vi "Esperienza 5 TEST 4F 4 paper.vi"() -> ()   [LabVIEW 2019]
uses:
  <vilib>/Analysis/baseanly.llb/Mean (DBL).vi
  <vilib>/Instr/_visa.llb/VISA Configure Serial Port (Instr).vi
  <vilib>/Utility/file.llb/Write Delimited Spreadsheet (DBL).vi
  <vilib>/Analysis/NI_AALBase.lvlib
panel:
  out "Ongoing":bool
  in  "IV":bool
  in  "Set Temperature Temperature":bool
  in  "Temperature Set":dbl=25.0 min=25.0 max=70.0 format="%#_6p"
  out "Actual temperature":dbl=25.0211735 caption="Temperature" format="%#.2g"
  out "V2":dbl[](graph)
  out "V1":dbl[](graph)
  out "V0":dbl[](graph)
  out "V2":dbl[](array[numeric])
  out "V1":dbl[](array[numeric])
  out "V0":dbl[](array[numeric])
  in  "R":dbl=10.0 format="%#_6p"
  out "Stabilization time":u8(slide)=3 scale=0.0..100.0
  in  "Skip stabilization?":bool
  in  "ITC ON?":bool=TRUE
  in  "Correction":i32=3000 min=0 max=4095 step=1
  in  "LED OP":u16(ring) items=["0.25 sun", "0.5 sun", "0.75 sun", "1 sun"]
  in  "number":i32=4095
  out "Actual current":dbl=0.005 caption="Temperature" format="%#_6p"
  out "Set":bool
  out "read buffer 2":string
  in  "File Name":string="Device 2.7"
  in  "file path":path=path "C:/Users/root/Desktop/Test Didattica Celle"
  in  "Save":bool
  in  "VISA ITC4005":refnum<visa-resource-name>="USB0::0x1313::0x804A::M00320668::INSTR" caption="resource name"
  out "IV Graph":cluster{"Y":dbl[], "Y":dbl[]}[](graph)=[{"Y"=[0.012, 0.023, 0.032, 0.044, 0.052, 0.068, 0.077, 0.085, 0.097, 0.108, 0.12, 0.131, 0.143, 0.152, 0.162, 0.175, 0.182, 0.196, 0.203, 0.218, 0.225, 0.24, 0.249, 0.259, 0.269, 0.281, 0.295, 0.302, 0.315, 0.322, 0.338, 0.348, 0.357, 0.367, 0.38, 0.39, 0.4, 0.409, 0.422, 0.433, 0.443, 0.453, 0.467, 0.476, 0.488, 0.496, 0.508, 0.518, 0.528, 0.537, 0.55, 0.559, 0.572, 0.582, 0.596, 0.6, 0.615, 0.623, 0.636, 0.648, 0.661, 0.67, 0.676, 0.691, 0.7, 0.716, 0.724, 0.732, 0.75, 0.753, 0.767, 0.778, 0.788, 0.799, 0.809, 0.82, 0.832, 0.843, 0.853, 0.862, 0.876, 0.885, 0.895, 0.905, 0.915, 0.929, 0.938, 0.95, 0.962, 0.973, 0.979, 0.99, 1.004, 1.012, 1.024, 1.035, 1.048, 1.058, 1.069, 1.077, 1.086, 1.098, 1.11, 1.12, 1.133, 1.144, 1.154, 1.161, 1.176, 1.184, 1.198, 1.207, 1.214, 1.227, 1.238, 1.248, 1.259, 1.273, 1.283, 1.293, 1.303, 1.315, 1.326, 1.335, 1.348, 1.356, 1.37, 1.378, 1.391, 1.401, 1.411, 1.421, 1.434, 1.443, 1.455, 1.464, 1.476, 1.487, 1.499, 1.509, 1.519, 1.53, 1.541, 1.551, 1.563, 1.572, 1.584, 1.596, 1.605, 1.615, 1.626, 1.638, 1.648, 1.657, 1.67, 1.68, 1.69, 1.701, 1.713, 1.722, 1.734, 1.744, 1.756, 1.766, 1.777, 1.787, 1.798, 1.809, 1.82, 1.831, 1.841, 1.852, 1.862, 1.873, 1.884, 1.895, 1.905, 1.917, 1.927, 1.937, 1.949, 1.958, 1.969, 1.979, 1.986, 1.99, 1.995, 1.999, 2.001, 2.006, 2.009, 2.013, 2.015, 2.018, 2.019, 2.023, 2.026, 2.027, 2.028, 2.032, 2.033, 2.035, 2.037, 2.038, 0.0], "Y"=[0.16, -0.08, -0.32, -0.24, 0.08, -0.08, 0.0, 0.0, 0.0, 0.0, 0.0, -0.16, -0.32, -0.08, -0.08, 0.0, 0.16, 0.0, 0.32, -0.24, 0.0, -0.24, -0.08, 0.08, 0.0, 0.0, -0.16, 0.08, -0.16, 0.32, 0.0, 0.32, 0.0, 0.16, -0.16, 0.16, 0.0, 0.4, 0.08, 0.24, 0.4, 0.08, 0.0, 0.0, 0.08, 0.24, 0.08, 0.0, 0.08, 0.24, 0.0, 0.24, 0.16, 0.24, -0.08, 0.48, 0.16, 0.24, 0.08, 0.24, 0.16, 0.08, 0.56, 0.24, 0.08, 0.16, 0.24, 0.24, -0.16, 0.32, 0.0, -0.16, 0.16, 0.16, 0.16, 0.32, 0.0, 0.16, 0.0, 0.24, 0.16, 0.16, 0.32, 0.48, 0.32, 0.16, 0.16, 0.08, 0.16, 0.24, 0.48, 0.48, 0.32, 0.4, 0.24, 0.16, 0.08, 0.24, 0.16, 0.48, 0.32, 0.56, 0.16, 0.48, 0.4, 0.16, 0.4, 0.48, 0.24, 0.48, 0.32, 0.56, 0.56, 0.64, 0.73, 0.81, 0.73, 0.73, 0.81, 0.64, 0.81, 1.05, 0.89, 0.81, 0.89, 0.97, 0.97, 1.05, 0.97, 1.21, 1.21, 1.13, 1.29, 1.45, 1.45, 1.53, 1.53, 1.53, 1.45, 1.61, 1.69, 1.77, 1.69, 1.85, 2.01, 2.01, 2.1, 2.18, 2.26, 2.42, 2.5, 2.58, 2.66, 2.66, 2.9, 2.9, 3.14, 3.14, 3.3, 3.3, 3.55, 3.63, 3.87, 4.03, 4.27, 4.43, 4.59, 4.59, 4.92, 5.0, 5.4, 5.56, 5.88, 6.12, 6.45, 6.77, 7.17, 7.41, 7.9, 8.22, 8.62, 9.11, 9.67, 9.91, 10.32, 10.64, 10.88, 11.12, 11.36, 11.52, 11.68, 11.85, 12.01, 12.25, 12.33, 12.57, 12.65, 12.81, 12.97, 13.05, 13.3, 13.46, 13.54, 13.7]}]
  out "I":dbl[](array[numeric])=[0.16, -0.08, -0.32, -0.24, 0.08, -0.08, 0.0, 0.0, 0.0, 0.0, 0.0, -0.16, -0.32, -0.08, -0.08, 0.0, 0.16, 0.0, 0.32, -0.24, 0.0, -0.24, -0.08, 0.08, 0.0, 0.0, -0.16, 0.08, -0.16, 0.32, 0.0, 0.32, 0.0, 0.16, -0.16, 0.16, 0.0, 0.4, 0.08, 0.24, 0.4, 0.08, 0.0, 0.0, 0.08, 0.24, 0.08, 0.0, 0.08, 0.24, 0.0, 0.24, 0.16, 0.24, -0.08, 0.48, 0.16, 0.24, 0.08, 0.24, 0.16, 0.08, 0.56, 0.24, 0.08, 0.16, 0.24, 0.24, -0.16, 0.32, 0.0, -0.16, 0.16, 0.16, 0.16, 0.32, 0.0, 0.16, 0.0, 0.24, 0.16, 0.16, 0.32, 0.48, 0.32, 0.16, 0.16, 0.08, 0.16, 0.24, 0.48, 0.48, 0.32, 0.4, 0.24, 0.16, 0.08, 0.24, 0.16, 0.48, 0.32, 0.56, 0.16, 0.48, 0.4, 0.16, 0.4, 0.48, 0.24, 0.48, 0.32, 0.56, 0.56, 0.64, 0.73, 0.8100000000000002, 0.73, 0.73, 0.8100000000000002, 0.64, 0.8100000000000002, 1.05, 0.89, 0.8100000000000002, 0.89, 0.97, 0.97, 1.05, 0.97, 1.21, 1.21, 1.13, 1.29, 1.45, 1.45, 1.53, 1.53, 1.53, 1.45, 1.61, 1.69, 1.77, 1.69, 1.85, 2.01, 2.01, 2.1, 2.18, 2.26, 2.42, 2.5, 2.58, 2.66, 2.66, 2.9, 2.9, 3.14, 3.14, 3.3, 3.3, 3.55, 3.63, 3.87, 4.03, 4.27, 4.43, 4.59, 4.59, 4.92, 5.0, 5.4, 5.56, 5.88, 6.12, 6.45, 6.769999999999999, 7.17, 7.409999999999999, 7.9, 8.22, 8.62, 9.11, 9.67, 9.91, 10.32, 10.64, 10.88, 11.12, 11.36, 11.52, 11.68, 11.85, 12.01, 12.25, 12.33, 12.57, 12.65, 12.809999999999999, 12.970000000000002, 13.05, 13.3, 13.460000000000003, 13.539999999999997, 13.7]
  out "V":dbl[](array[numeric])=[0.012, 0.023, 0.032, 0.044, 0.052, 0.068, 0.077, 0.085, 0.097, 0.108, 0.12, 0.131, 0.143, 0.152, 0.162, 0.175, 0.182, 0.196, 0.203, 0.218, 0.225, 0.24, 0.249, 0.259, 0.269, 0.281, 0.295, 0.302, 0.315, 0.322, 0.338, 0.348, 0.357, 0.367, 0.38, 0.39, 0.4, 0.409, 0.422, 0.433, 0.443, 0.453, 0.467, 0.476, 0.488, 0.496, 0.508, 0.518, 0.528, 0.537, 0.55, 0.559, 0.572, 0.582, 0.596, 0.6, 0.615, 0.623, 0.636, 0.648, 0.661, 0.67, 0.676, 0.691, 0.7, 0.716, 0.724, 0.732, 0.75, 0.753, 0.767, 0.778, 0.788, 0.799, 0.809, 0.82, 0.832, 0.843, 0.853, 0.862, 0.876, 0.885, 0.895, 0.905, 0.915, 0.929, 0.938, 0.95, 0.962, 0.973, 0.979, 0.99, 1.004, 1.012, 1.024, 1.035, 1.048, 1.058, 1.069, 1.077, 1.086, 1.098, 1.11, 1.12, 1.133, 1.144, 1.154, 1.161, 1.176, 1.184, 1.198, 1.207, 1.214, 1.227, 1.238, 1.248, 1.259, 1.273, 1.283, 1.293, 1.303, 1.315, 1.326, 1.335, 1.348, 1.356, 1.37, 1.378, 1.391, 1.401, 1.411, 1.421, 1.434, 1.443, 1.455, 1.464, 1.476, 1.487, 1.499, 1.509, 1.519, 1.53, 1.541, 1.551, 1.563, 1.572, 1.584, 1.596, 1.605, 1.615, 1.626, 1.638, 1.648, 1.657, 1.67, 1.68, 1.69, 1.701, 1.713, 1.722, 1.734, 1.744, 1.756, 1.766, 1.777, 1.787, 1.798, 1.809, 1.82, 1.831, 1.841, 1.852, 1.862, 1.873, 1.884, 1.895, 1.905, 1.917, 1.927, 1.937, 1.949, 1.958, 1.969, 1.979, 1.986, 1.99, 1.995, 1.999, 2.001, 2.006, 2.009, 2.013, 2.015, 2.018, 2.019, 2.023, 2.026, 2.027, 2.028, 2.032, 2.033, 2.035, 2.037, 2.038, 0.0]
  out "array":dbl[](array[numeric])=[0.053, 0.08, 0.012, 0.16, 0.023, -0.08, 0.032, -0.32, 0.044, -0.24, 0.052, 0.08, 0.068, -0.08, 0.077, 0.0, 0.085, 0.0, 0.097, 0.0, 0.108, 0.0, 0.12, 0.0, 0.131, -0.16, 0.143, -0.32, 0.152, -0.08, 0.162, -0.08, 0.175, 0.0, 0.182, 0.16, 0.196, 0.0, 0.203, 0.32, 0.218, -0.24, 0.225, 0.0, 0.24, -0.24, 0.249, -0.08, 0.259, 0.08, 0.269, 0.0, 0.281, 0.0, 0.295, -0.16, 0.302, 0.08, 0.315, -0.16, 0.322, 0.32, 0.338, 0.0, 0.348, 0.32, 0.357, 0.0, 0.367, 0.16, 0.38, -0.16, 0.39, 0.16, 0.4, 0.0, 0.409, 0.4, 0.422, 0.08, 0.433, 0.24, 0.443, 0.4, 0.453, 0.08, 0.467, 0.0, 0.476, 0.0, 0.488, 0.08, 0.496, 0.24, 0.508, 0.08, 0.518, 0.0, 0.528, 0.08, 0.537, 0.24, 0.55, 0.0, 0.559, 0.24, 0.572, 0.16, 0.582, 0.24, 0.596, -0.08, 0.6, 0.48, 0.615, 0.16, 0.623, 0.24, 0.636, 0.08, 0.648, 0.24, 0.661, 0.16, 0.67, 0.08, 0.676, 0.56, 0.691, 0.24, 0.7, 0.08, 0.716, 0.16, 0.724, 0.24, 0.732, 0.24, 0.75, -0.16, 0.753, 0.32, 0.767, 0.0, 0.778, -0.16, 0.788, 0.16, 0.799, 0.16, 0.809, 0.16, 0.82, 0.32, 0.832, 0.0, 0.843, 0.16, 0.853, 0.0, 0.862, 0.24, 0.876, 0.16, 0.885, 0.16, 0.895, 0.32, 0.905, 0.48, 0.915, 0.32, 0.929, 0.16, 0.938, 0.16, 0.95, 0.08, 0.962, 0.16, 0.973, 0.24, 0.979, 0.48, 0.99, 0.48, 1.004, 0.32, 1.012, 0.4, 1.024, 0.24, 1.035, 0.16, 1.048, 0.08, 1.058, 0.24, 1.069, 0.16, 1.077, 0.48, 1.086, 0.32, 1.098, 0.56, 1.11, 0.16, 1.12, 0.48, 1.133, 0.4, 1.144, 0.16, 1.154, 0.4, 1.161, 0.48, 1.176, 0.24, 1.184, 0.48, 1.198, 0.32, 1.207, 0.56, 1.214, 0.56, 1.227, 0.64, 1.238, 0.73, 1.248, 0.81, 1.259, 0.73, 1.273, 0.73, 1.283, 0.81, 1.293, 0.64, 1.303, 0.81, 1.315, 1.05, 1.326, 0.89, 1.335, 0.81, 1.348, 0.89, 1.356, 0.97, 1.37, 0.97, 1.378, 1.05, 1.391, 0.97, 1.401, 1.21, 1.411, 1.21, 1.421, 1.13, 1.434, 1.29, 1.443, 1.45, 1.455, 1.45, 1.464, 1.53, 1.476, 1.53, 1.487, 1.53, 1.499, 1.45, 1.509, 1.61, 1.519, 1.69, 1.53, 1.77, 1.541, 1.69, 1.551, 1.85, 1.563, 2.01, 1.572, 2.01, 1.584, 2.1, 1.596, 2.18, 1.605, 2.26, 1.615, 2.42, 1.626, 2.5, 1.638, 2.58, 1.648, 2.66, 1.657, 2.66, 1.67, 2.9, 1.68, 2.9, 1.69, 3.14, 1.701, 3.14, 1.713, 3.3, 1.722, 3.3, 1.734, 3.55, 1.744, 3.63, 1.756, 3.87, 1.766, 4.03, 1.777, 4.27, 1.787, 4.43, 1.798, 4.59, 1.809, 4.59, 1.82, 4.92, 1.831, 5.0, 1.841, 5.4, 1.852, 5.56, 1.862, 5.88, 1.873, 6.12, 1.884, 6.45, 1.895, 6.77, 1.905, 7.17, 1.917, 7.41, 1.927, 7.9, 1.937, 8.22, 1.949, 8.62, 1.958, 9.11, 1.969, 9.67, 1.979, 9.91, 1.986, 10.32, 1.99, 10.64, 1.995, 10.88, 1.999, 11.12, 2.001, 11.36, 2.006, 11.52, 2.009, 11.68, 2.013, 11.85, 2.015, 12.01, 2.018, 12.25, 2.019, 12.33, 2.023, 12.57, 2.026, 12.65, 2.027, 12.81, 2.028, 12.97, 2.032, 13.05, 2.033, 13.3, 2.035, 13.46, 2.037, 13.54, 2.038, 13.7, 0.0]
  out "read buffer":string="LED OFF\r\n"
  in  "Arduino":refnum<visa-resource-name>="COM3"
  in  "Set LED Current":bool
  in  "LED Current":dbl=0.005 min=0.005 max=0.02 format="%#_6p"
  out "error out":errorcluster={"status"=FALSE, "code"=1073676294, "source"=""}
  in  "Abort Program":bool
  in  "LED":bool
  # "CONFIGURATION"
  # "LED CONTROL"
  # "MEASUREMENT"
  # "TEMPERATURE\nCONTROL"
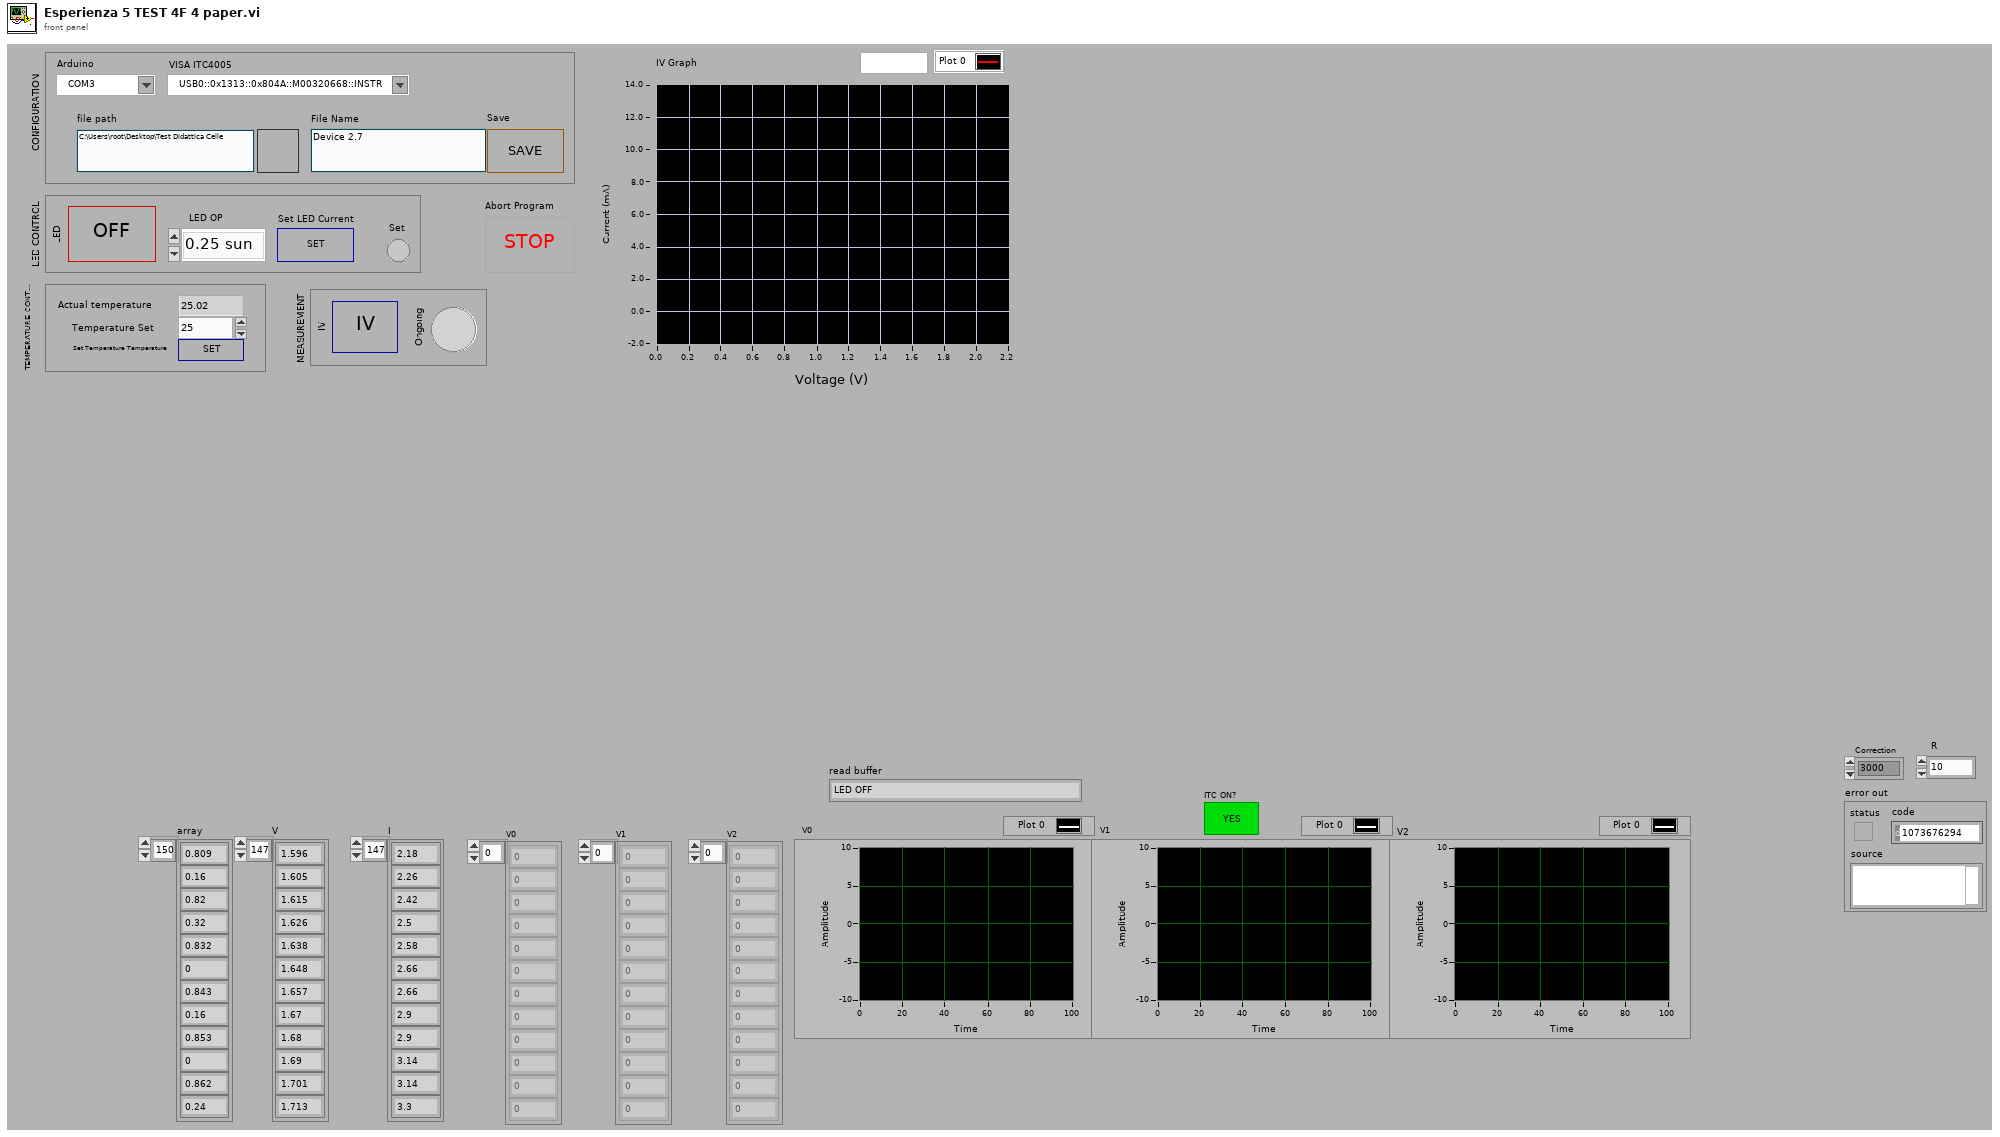
[diagram p1: front panel]
types:
  T1 = cluster{"TEC Operating Mode (Constant Temperature)":i16, "TEC Temperature Setpoint (20.0)":dbl}
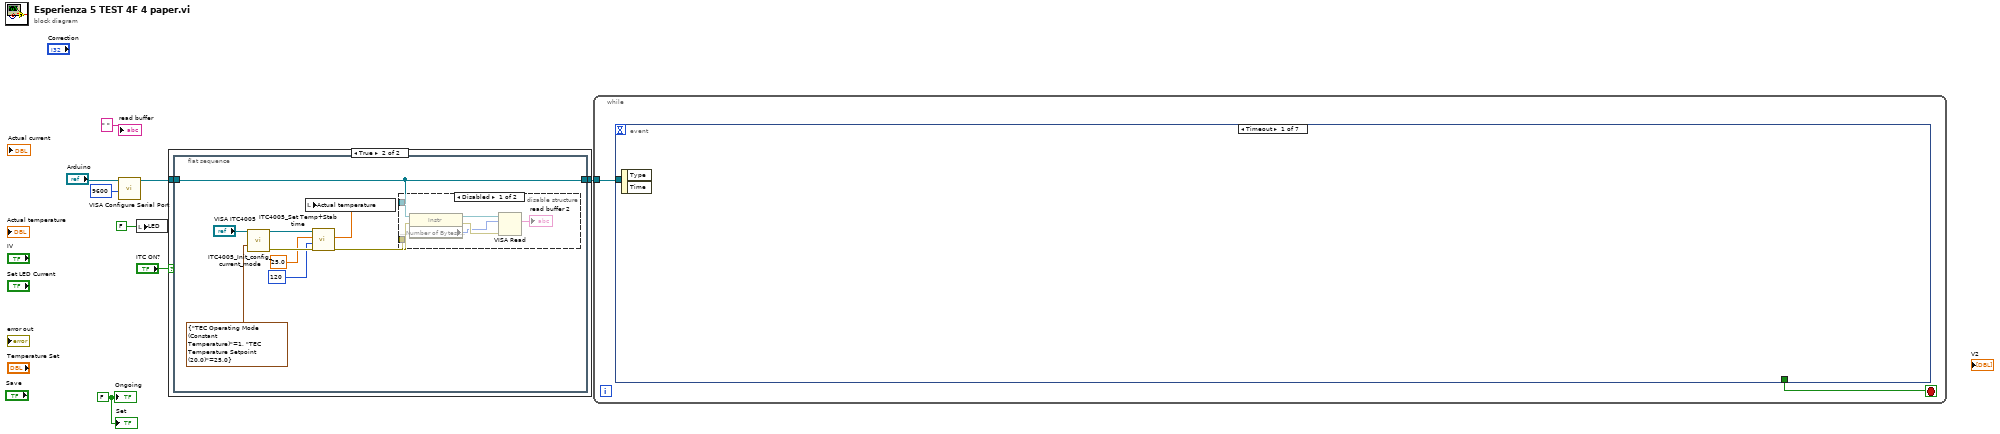
[diagram p0: block diagram]
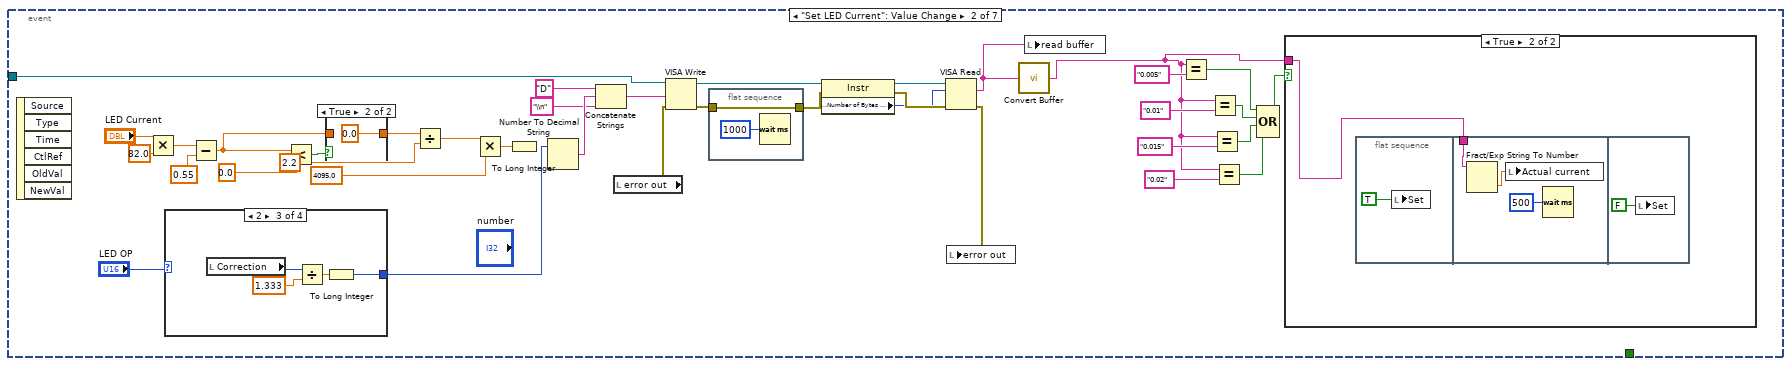
[diagram p4: hidden frame]
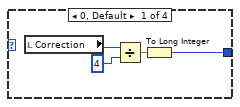
[diagram p5: hidden frame]
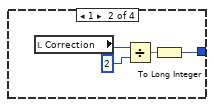
[diagram p6: hidden frame]
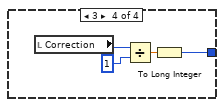
[diagram p7: hidden frame]
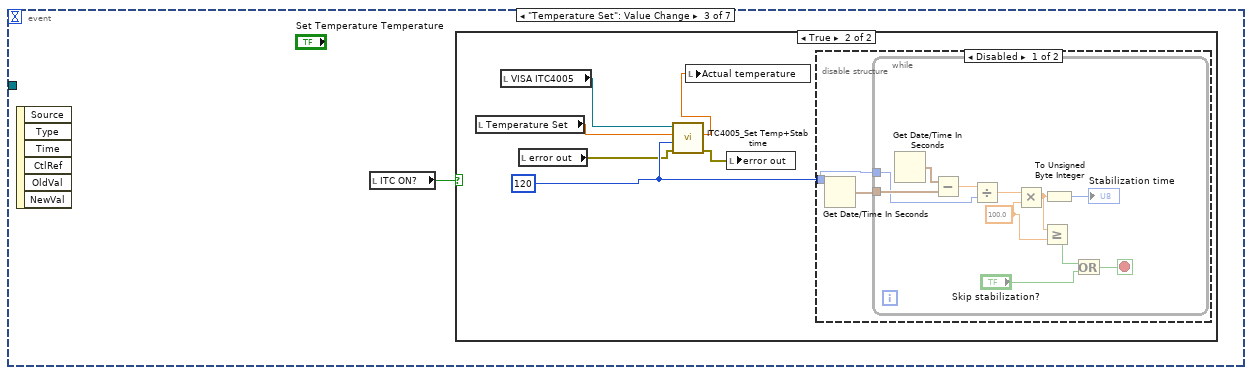
[diagram p10: hidden frame]
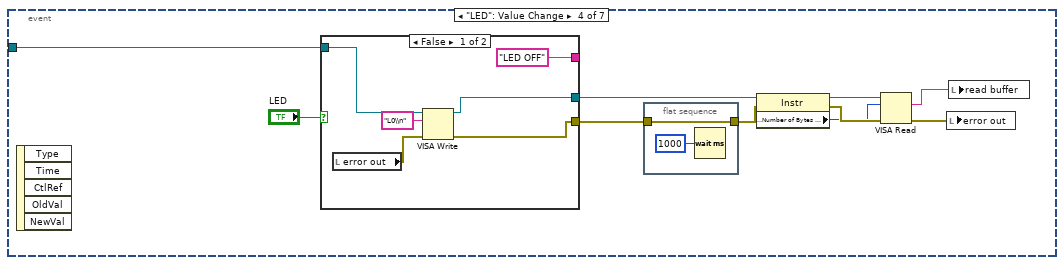
[diagram p13: hidden frame]
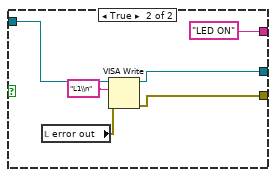
[diagram p14: hidden frame]
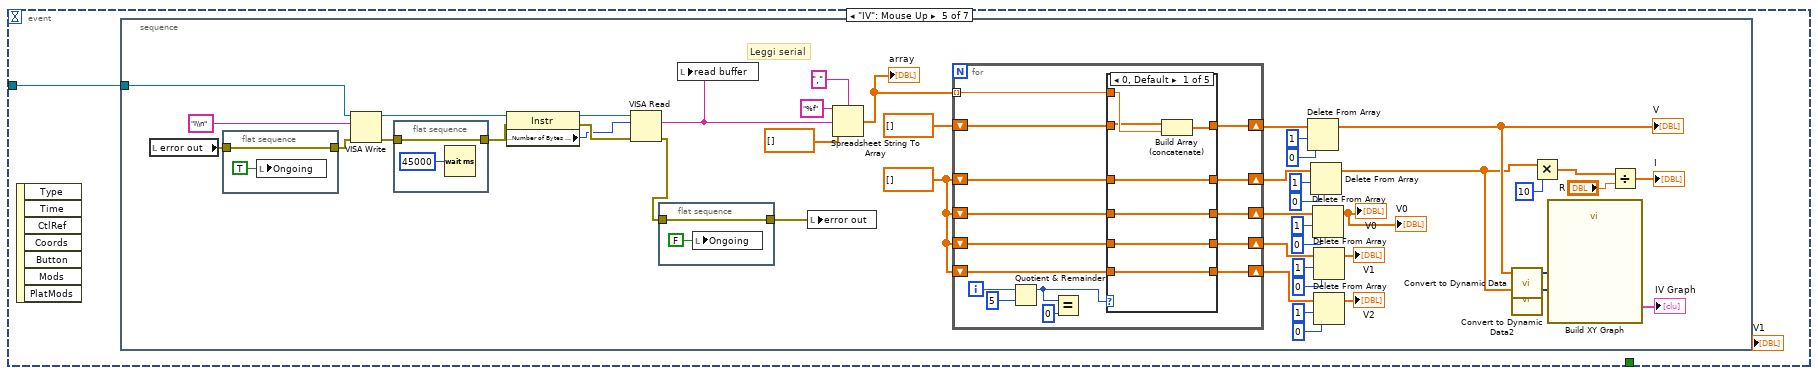
[diagram p15: hidden frame]
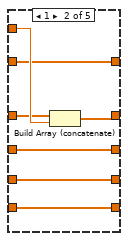
[diagram p16: hidden frame]
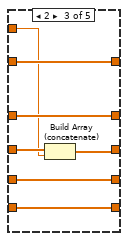
[diagram p17: hidden frame]
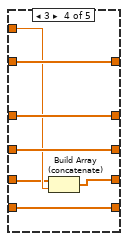
[diagram p18: hidden frame]
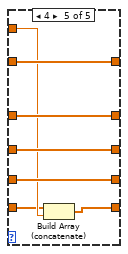
[diagram p19: hidden frame]
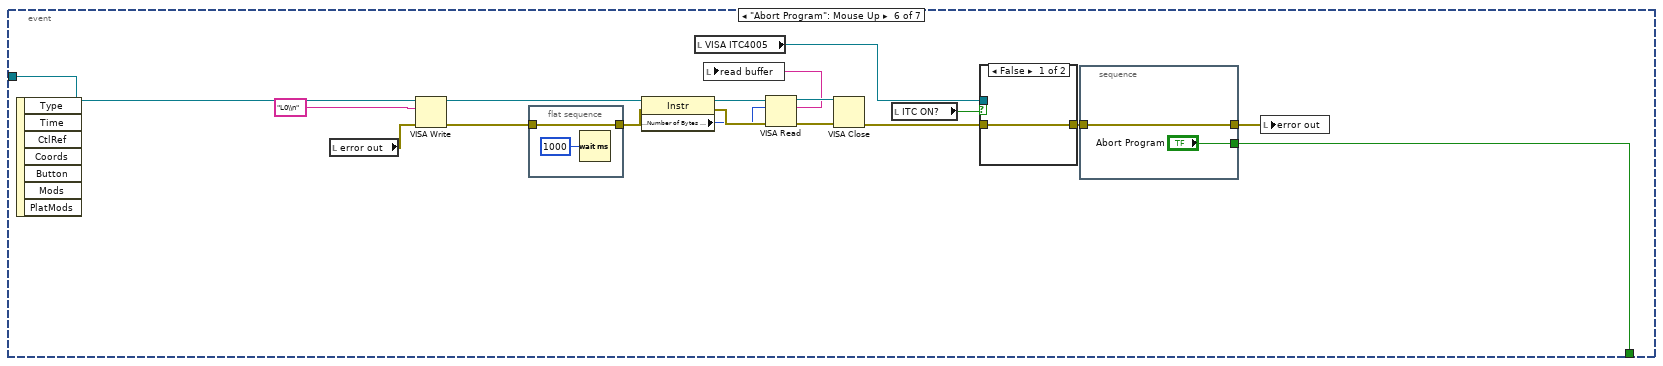
[diagram p20: hidden frame]
diagram:
  w2 = FALSE ("Ongoing")
  n1 = call-poly "VISA Configure Serial Port"("VISA resource name"="Arduino", "baud rate (9600)"=u32 9600) -> ("VISA resource name out"=w3:refnum<visa-resource-name>)  [unwired: 12 in, 1 out]
  n2 = local write "LED"(FALSE ("LED")) -> ()
  n3 = case shown="True" "ITC ON?" {
    tunnel: [w9 w11] -> w4
    tunnel: w3 -> [w9 w10]
    frame False {
    }
    frame True {
      n4 = flat-sequence {
        tunnel: [w14] -> w11
        tunnel: w10 -> [w14]
        frame #0 {
          n5 = call "ITC4005_Init_config_current_mode.vi"("VISA ITC4005"="VISA ITC4005", "TEC Settings"=T1 {"TEC Operating Mode (Constant Temperature)"=1, "TEC Temperature Setpoint (20.0)"=25.0}) -> ("ITC4005 handle out"=w19:refnum<visa-resource-name>, "error out"=w18:errorcluster)  [unwired: 12 in]
          n6 = call "ITC4005_Set Temp+Stab time.vi"("error in"=w18, "Stabilization Time (s)"=120, "TEC Temperature Setpoint (20.0)"=25.0, "ITC4005 handle in"=w19) -> ("error out"=w13:errorcluster, "Actual temperature"=w12:dbl)  [unwired: 4 in, 2 out]
          n7 = local write "Actual temperature"(w12) -> ()
          n8 = disable-structure shown="Disabled" {
            disable-tunnel: w14 -> [w23 _]
            disable-tunnel: w13 -> [w22 _]
            frame Disabled {
              n9 = property class="Instr"(reference=w23, error in=w22) -> (reference out=w25:refnum<visa-resource-name>, error out=w26:errorcluster, "Serial Settings:Number of Bytes at Serial Port"=w24:u32)
              n10 = VISA Read(VISA resource name=w25, byte count=w24, error in (no error)=w26) -> (read buffer=→"read buffer 2":string)  [unwired: 3 out]
            }
            frame Enabled {
            }
          }
        }
      }
    }
  }
  n11 = while {
    tunnel: w4 -> [w28]
    stop <- w27 stop-if-true
    n12 = event shown="[0] Timeout" {
      selector: _ -> [_ _ _ _ _ _ _]
      dyn-events: _ -> [_ _ _ _ _ _ _]
      timeout: _ -> [_ _ _ _ _ _ _]
      tunnel: w28 -> [_ w51 _ w122 w137 w256 _]
      tunnel: [_ _ _ _ _ w245 _] -> w27
      event Timeout {
        n13 = event-data() -> ()  [unwired: 1 in, 2 out]
      }
      event "Set LED Current": Value Change {
        n14 = event-data() -> ()  [unwired: 1 in, 6 out]
        n15 = Multiply(x="LED Current", y=82.0) -> (x*y=w64:dbl)
        n16 = case shown="2" "LED OP" {
          tunnel: [w68 w71 w75 w79] -> w29
          frame 0, Default {
            n17 = local read "Correction"() -> (w70:i32)
            n18 = Divide(x=w70, y=4) -> (x/y=w69:dbl)
            n19 = To Long Integer(number=w69) -> (32bit integer=w68:i32)
          }
          frame 1 {
            n20 = local read "Correction"() -> (w74:i32)
            n21 = Divide(x=w74, y=2) -> (x/y=w73:dbl)
            n22 = To Long Integer(number=w73) -> (32bit integer=w71:i32)
          }
          frame 2 {
            n23 = local read "Correction"() -> (w78:i32)
            n24 = Divide(x=w78, y=1.333) -> (x/y=w77:dbl)
            n25 = To Long Integer(number=w77) -> (32bit integer=w75:i32)
          }
          frame 3 {
            n26 = local read "Correction"() -> (w82:i32)
            n27 = Divide(x=w82, y=1) -> (x/y=w81:dbl)
            n28 = To Long Integer(number=w81) -> (32bit integer=w79:i32)
          }
        }
        n29 = Subtract(x=w64, y=0.55) -> (x-y=w60:dbl)
        n30 = Less?(x=w60, y=0.0) -> (x < y?=w61:bool)
        n31 = case shown="True" w61 {
          tunnel: [w91 0.0 ("y")] -> w59
          tunnel: w60 -> [w91 _]
          frame False {
          }
          frame True {
          }
        }
        n32 = Divide(x=w59, y=2.2) -> (x/y=w57:dbl)
        n33 = Multiply(x=w57, y=4095.0) -> (x*y=w55:dbl)
        n34 = To Long Integer(number=w55) -> ()  [unwired: 1 out]
        n35 = Number To Decimal String(number=w29) -> (decimal integer string=w54:string)  [unwired: 1 in]
        n36 = Concatenate Strings("D" ("string"), w54, "\\n" ("string")) -> (w52:string)
        n37 = local read "error out"() -> (w50:errorcluster)
        n38 = VISA Write(VISA resource name=w51, write buffer=w52, error in (no error)=w50) -> (VISA resource name out=w44:refnum<visa-resource-name>, error out=w42:errorcluster)  [unwired: 1 out]
        n39 = flat-sequence {
          tunnel: w42 -> [w89]
          tunnel: [w89] -> w48
          frame #0 {
            n40 = Wait (ms)(milliseconds to wait=u32 1000) -> ()  [unwired: 1 out]
          }
        }
        n41 = property class="Instr"(reference=w44, error in=w48) -> (reference out=w46:refnum<visa-resource-name>, error out=w47:errorcluster, "Serial Settings:Number of Bytes at Serial Port"=w45:u32)
        n42 = VISA Read(VISA resource name=w46, byte count=w45, error in (no error)=w47) -> (read buffer=w32:string, error out=w43:errorcluster)  [unwired: 2 out]
        n43 = local write "error out"(w43) -> ()
        n44 = call "Convert Buffer.vi"("Buffer"=w32) -> ("Out String"=w31:string)
        n45 = local write "read buffer"(w32) -> ()
        n46 = Equal?(x=w31, y="0.005") -> (x = y?=w37:bool)
        n47 = Equal?(x=w31, y="0.01") -> (x = y?=w36:bool)
        n48 = Equal?(x=w31, y="0.015") -> (x = y?=w35:bool)
        n49 = Equal?(x=w31, y="0.02") -> (x = y?=w34:bool)
        n50 = Compound Arithmetic op=OR(w37, w36, w35, w34) -> (w33:bool)
        n51 = case shown="True" w33 {
          tunnel: w31 -> [_ w83]
          frame False {
          }
          frame True {
            n52 = flat-sequence {
              tunnel: w83 -> [w86]
              frame #0 {
                n53 = local write "Set"(TRUE ("Setted")) -> ()
              }
              frame #1 {
                n54 = Fract/Exp String To Number(string=w86) -> (number=w85:dbl)  [unwired: 3 in, 1 out]
                n55 = local write "Actual current"(w85) -> ()
                n56 = Wait (ms)(milliseconds to wait=u32 500) -> ()  [unwired: 1 out]
              }
              frame #2 {
                n57 = local write "Set"(FALSE ("Setted")) -> ()
              }
            }
          }
        }
      }
      event "Temperature Set": Value Change {
        n58 = event-data() -> ()  [unwired: 1 in, 6 out]
        n59 = local read "ITC ON?"() -> (w93:bool)
        n60 = case shown="True" w93 {
          frame False {
          }
          frame True {
            w99 = 120 ("Stabilization Time (s)")
            n61 = local read "Temperature Set"() -> (w97:dbl)
            n62 = local read "VISA ITC4005"() -> (w98:refnum<visa-resource-name>)
            n63 = local read "error out"() -> (w96:errorcluster)
            n64 = call "ITC4005_Set Temp+Stab time.vi"("error in"=w96, "Stabilization Time (s)"=w99, "TEC Temperature Setpoint (20.0)"=w97, "ITC4005 handle in"=w98) -> ("error out"=w95:errorcluster, "Actual temperature"=w94:dbl)  [unwired: 4 in, 2 out]
            n65 = local write "Actual temperature"(w94) -> ()
            n66 = local write "error out"(w95) -> ()
            n67 = disable-structure shown="Disabled" {
              disable-tunnel: w99 -> [w101 _]
              frame Disabled {
                n68 = Get Date/Time In Seconds() -> (seconds since 1Jan1904=w100:timestamp)
                n69 = while {
                  tunnel: w100 -> [w112]
                  tunnel: w101 -> [w109]
                  stop <- w104 stop-if-true
                  w106 = 100.0 ("y")
                  n70 = Get Date/Time In Seconds() -> (seconds since 1Jan1904=w111:timestamp)
                  n71 = Subtract(x=w111, y=w112) -> (x-y=w110:dbl)
                  n72 = Divide(x=w110, y=w109) -> (x/y=w108:dbl)
                  n73 = Multiply(x=w108, y=w106) -> (x*y=w107:dbl)
                  n74 = Greater Or Equal?(x=w107, y=w106) -> (x >= y?=w105:bool)
                  n75 = To Unsigned Byte Integer(number=w107) -> (unsigned 8bit integer=→"Stabilization time":u8)
                  n76 = Or(x=w105, y="Skip stabilization?") -> (x .or. y?=w104:bool)
                }
              }
              frame Enabled {
              }
            }
          }
        }
      }
      event "LED": Value Change {
        n77 = event-data() -> ()  [unwired: 1 in, 5 out]
        n78 = case shown="False" "LED" {
          tunnel: w122 -> [w129 w135]
          tunnel: [w126 w133] -> w115
          tunnel: [w127 w132] -> w114
          tunnel: ["LED OFF" ("write buffer") "LED ON" ("write buffer")] -> _
          frame False {
            n79 = local read "error out"() -> (w128:errorcluster)
            n80 = VISA Write(VISA resource name=w129, write buffer="L0\\n", error in (no error)=w128) -> (VISA resource name out=w127:refnum<visa-resource-name>, error out=w126:errorcluster)  [unwired: 1 out]
          }
          frame True {
            n81 = local read "error out"() -> (w134:errorcluster)
            n82 = VISA Write(VISA resource name=w135, write buffer="L1\\n", error in (no error)=w134) -> (VISA resource name out=w132:refnum<visa-resource-name>, error out=w133:errorcluster)  [unwired: 1 out]
          }
        }
        n83 = flat-sequence {
          tunnel: w115 -> [w123]
          tunnel: [w123] -> w120
          frame #0 {
            n84 = Wait (ms)(milliseconds to wait=u32 1000) -> ()  [unwired: 1 out]
          }
        }
        n85 = property class="Instr"(reference=w114, error in=w120) -> (reference out=w118:refnum<visa-resource-name>, error out=w119:errorcluster, "Serial Settings:Number of Bytes at Serial Port"=w117:u32)
        n86 = VISA Read(VISA resource name=w118, byte count=w117, error in (no error)=w119) -> (read buffer=w113:string, error out=w116:errorcluster)  [unwired: 2 out]
        n87 = local write "error out"(w116) -> ()
        n88 = local write "read buffer"(w113) -> ()
      }
      event "IV": Mouse Up {
        n89 = event-data() -> ()  [unwired: 1 in, 7 out]
        n90 = stacked-sequence {
          tunnel: w137 -> [w177]
          frame #0 {
            w150 = dbl[] []
            # "Leggi serial"
            n91 = local read "error out"() -> (w160:errorcluster)
            n92 = flat-sequence {
              tunnel: [w187] -> w161
              tunnel: w160 -> [w187]
              frame #0 {
                n93 = local write "Ongoing"(TRUE ("Ongoing")) -> ()
              }
            }
            n94 = VISA Write(VISA resource name=w177, write buffer="I\\n", error in (no error)=w161) -> (VISA resource name out=w179:refnum<visa-resource-name>, error out=w182:errorcluster)  [unwired: 1 out]
            n95 = flat-sequence {
              tunnel: w182 -> [w238]
              tunnel: [w238] -> w181
              frame #0 {
                n96 = Wait (ms)(milliseconds to wait=u32 45000) -> ()  [unwired: 1 out]
              }
            }
            n97 = property class="Instr"(reference=w179, error in=w181) -> (reference out=w178:refnum<visa-resource-name>, error out=w180:errorcluster, "Serial Settings:Number of Bytes at Serial Port"=w156:u32)
            n98 = VISA Read(VISA resource name=w178, byte count=w156, error in (no error)=w180) -> (read buffer=w162:string, error out=w158:errorcluster)  [unwired: 2 out]
            n99 = flat-sequence {
              tunnel: [w185] -> w157
              tunnel: w158 -> [w185]
              frame #0 {
                n100 = local write "Ongoing"(FALSE ("Ongoing")) -> ()
              }
            }
            n101 = local write "read buffer"(w162) -> ()
            n102 = local write "error out"(w157) -> ()
            n103 = Spreadsheet String To Array(delimiter (Tab)=",", format string="%f", spreadsheet string=w162, array type (2D Dbl)=dbl[] []) -> (array=w163:dbl[])
            "array" <- w163
            n104 = for {
              tunnel: w163 -> [w199] mode=indexing
              shift-right: [w197] -> w169
              shift-left: dbl[] [] -> [w198]
              shift-right: [w195] -> w164
              shift-left: w150 -> [w196]
              shift-right: [w192] -> w141
              shift-left: w150 -> [w193]
              shift-right: [w190] -> w142
              shift-left: w150 -> [w191]
              shift-right: [w188] -> w143
              shift-left: w150 -> [w189]
              i -> [w202]
              n105 = Quotient & Remainder(x=w202, y=5) -> (x-y*floor(x/y)=w194:i32)  [unwired: 1 out]
              n106 = Equal?(x=w194, y=0) -> ()  [unwired: 1 out]
              n107 = case shown="0, Default" w194 {
                tunnel: w199 -> [w209 w216 w217 w226 w233]
                tunnel: w198 -> [w207 w213 w223 w230 w237]
                tunnel: [w208 w213 w223 w230 w237] -> w197
                tunnel: w196 -> [w206 w215 w222 w229 w236]
                tunnel: [w206 w214 w222 w229 w236] -> w195
                tunnel: w193 -> [w205 w212 w219 w228 w235]
                tunnel: [w205 w212 w218 w228 w235] -> w192
                tunnel: w191 -> [w204 w211 w221 w225 w234]
                tunnel: [w204 w211 w221 w224 w234] -> w190
                tunnel: w189 -> [w203 w210 w220 w227 w232]
                tunnel: [w203 w210 w220 w227 w231] -> w188
                frame 0, Default {
                  n108 = Build Array (concatenate)(w207, w209) -> (w208:dbl[])
                }
                frame 1 {
                  n109 = Build Array (concatenate)(w215, w216) -> (w214:dbl[])
                }
                frame 2 {
                  n110 = Build Array (concatenate)(w219, w217) -> (w218:dbl[])
                }
                frame 3 {
                  n111 = Build Array (concatenate)(w225, w226) -> (w224:dbl[])
                }
                frame 4 {
                  n112 = Build Array (concatenate)(w232, w233) -> (w231:dbl[])
                }
              }
            }
            n113 = Delete From Array(array=w169, length=1, index=0) -> (array with subset deleted=w159:dbl[])  [unwired: 1 out]
            "V" <- w159
            n114 = Delete From Array(array=w164, length=1, index=0) -> (array with subset deleted=w154:dbl[])  [unwired: 1 out]
            n115 = Delete From Array(array=w141, length=1, index=0) -> (array with subset deleted=→"V0" →"V0":dbl[])  [unwired: 1 out]
            n116 = Delete From Array(array=w142, length=1, index=0) -> (array with subset deleted=→"V1":dbl[])  [unwired: 1 out]
            n117 = Delete From Array(array=w143, length=1, index=0) -> (array with subset deleted=→"V2":dbl[])  [unwired: 1 out]
            n118 = call "Convert to Dynamic Data"("Array"=w159) -> ("Dynamic Data Type"=w171:dynamicdata)  [unwired: 3 in]
            n119 = call "Convert to Dynamic Data2"("Array"=w154) -> ("Dynamic Data Type"=w170:dynamicdata)  [unwired: 3 in]
            n120 = Multiply(x=w154, y=10) -> (x*y=w155:dbl[])
            n121 = call "Build XY Graph"("Y Input"=w170, "X Input"=w171) -> ("XY Graph"=→"IV Graph":cluster{"Y":dbl[], "Y":dbl[]}[])  [unwired: 8 in, 1 out]
            n122 = Divide(x=w155, y="R") -> (x/y=→"I":dbl[])
          }
        }
      }
      event "Abort Program": Mouse Up {
        n123 = event-data() -> ()  [unwired: 1 in, 7 out]
        n124 = local read "error out"() -> (w255:errorcluster)
        n125 = VISA Write(VISA resource name=w256, write buffer="L0\\n", error in (no error)=w255) -> (VISA resource name out=w249:refnum<visa-resource-name>, error out=w248:errorcluster)  [unwired: 1 out]
        n126 = flat-sequence {
          tunnel: w248 -> [w265]
          tunnel: [w265] -> w254
          frame #0 {
            n127 = Wait (ms)(milliseconds to wait=u32 1000) -> ()  [unwired: 1 out]
          }
        }
        n128 = property class="Instr"(reference=w249, error in=w254) -> (reference out=w252:refnum<visa-resource-name>, error out=w253:errorcluster, "Serial Settings:Number of Bytes at Serial Port"=w251:u32)
        n129 = local read "VISA ITC4005"() -> (w241:refnum<visa-resource-name>)
        n130 = VISA Read(VISA resource name=w252, byte count=w251, error in (no error)=w253) -> (VISA resource name out=w250:refnum<visa-resource-name>, read buffer=w244:string, error out=w247:errorcluster)  [unwired: 1 out]
        n131 = local write "read buffer"(w244) -> ()
        n132 = VISA Close(VISA resource name=w250, error in (no error)=w247) -> (error out=w243:errorcluster)
        n133 = local read "ITC ON?"() -> (w240:bool)
        n134 = case shown="False" w240 {
          tunnel: w243 -> [w258 w262]
          tunnel: [w258 w261] -> w242
          tunnel: w241 -> [_ w260]
          frame False {
          }
          frame True {
            n135 = call "TL4000 Switch TEC Output.vi"("error in (no error)"=w262, "TEC Output (Off)"=FALSE, "instrument handle"=w260) -> ("error out"=w261:errorcluster)  [unwired: 7 in, 1 out]
          }
        }
        n136 = stacked-sequence {
          tunnel: w242 -> [w264]
          tunnel: [w264] -> w246
          tunnel: ["Abort Program"] -> w245
          frame #0 {
          }
        }
        n137 = local write "error out"(w246) -> ()
      }
      event "Save": Mouse Up {
        n138 = event-data() -> ()  [unwired: 1 in, 8 out]
        n139 = local read "V"() -> (w275:dbl[])
        n140 = local read "I"() -> (w278:dbl[])
        n141 = Array Size(array=w278) -> (size(s)=w272:i32)
        n142 = Array Size(array=w275) -> (size(s)=w268:i32)
        n143 = Array Subset(array=w278, index=0, length=3) -> (w283:dbl[])
        n144 = Subtract(x=w272, y=0) -> (x-y=w271:i32)
        n145 = Subtract(x=w268, y=1) -> (x-y=w267:i32)
        n146 = Delete From Array(array=w278, length=0, index=w271) -> (array with subset deleted=w277:dbl[])  [unwired: 1 out]
        n147 = Delete From Array(array=w275, length=1, index=w267) -> (array with subset deleted=w276:dbl[])  [unwired: 1 out]
        n148 = call-poly <vilib>:"Mean.vi"("X"=w283) -> ("mean"=w282:dbl)  [unwired: 1 out]
        n149 = Build Array (concatenate)(w282, w277) -> (w281:dbl[])
        n150 = Build Array (concatenate)(0.0 ("y"), w276) -> (w280:dbl[])
        n151 = Build Array(w280, w281) -> (w294:dbl[][])
        n152 = Concatenate Strings("File Name", ".txt" ("string")) -> (w288:string)
        n153 = Build Path(base path="file path", name or relative path=w288) -> (appended path=w290:path)
        n154 = call-poly <vilib>:"Write Delimited Spreadsheet.vi"("file path (dialog if empty)"=w290, "format (%.3f)"="%.3f", "2D data"=w294, "append to file? (new file:F)"=TRUE, "transpose? (no:F)"=TRUE) -> ()  [unwired: 9 in, 2 out]
      }
    }
  }
  "read buffer" <- " " ("read buffer")
  "Ongoing" <- w2
  "Set" <- w2
